vi "Write Last Result.vi"(10 "Result":refnum<class "Result.lvclass">, 11 "Results in":refnum<class "Results.lvclass">) -> (3 "Results out":refnum<class "Results.lvclass">)   [LabVIEW 2018, in "InfluxDB Client.lvlib" / "Results.lvclass"]
uses:
  Results.lvclass
  Result/Result.lvclass
  Results.lvclass/Results.ctl
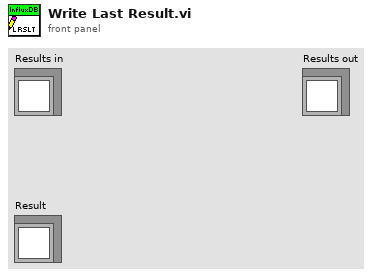
[diagram p1: front panel]
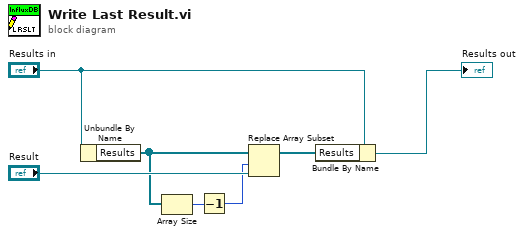
[diagram p0: block diagram]
diagram:
  n1 = Unbundle By Name("Results in") -> ("Results"=w3:refnum<class "Result.lvclass">[])
  n2 = Array Size(array=w3) -> (size(s)=w2:i32)
  n3 = Decrement(x=w2) -> (x-1=w1:i32)
  n4 = Replace Array Subset(array=w3, new element="Result", index=w1) -> (w4:refnum<class "Result.lvclass">[])
  n5 = Bundle By Name(cluster="Results in", "Results"=w4) -> (→"Results out":refnum<class "Results.lvclass">)
